vi "Set loggingEnabled.vi"(8 "error in (no error)":errorcluster, 10 "loggingEnabled":bool=TRUE, 11 "niDTS Comm String in":refnum<class "niDTS Comm String.lvclass">) -> (0 "error out":errorcluster, 3 "niDTS Comm String out":refnum<class "niDTS Comm String.lvclass">)   [LabVIEW 2015, in "niDTS CommLib.lvlib" / "niDTS Comm String.lvclass"]
uses:
  niDTS Comm String.lvclass
  niDTS Comm String.lvclass/niDTS Comm String.ctl
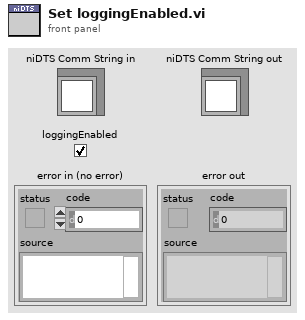
[diagram p1: front panel]
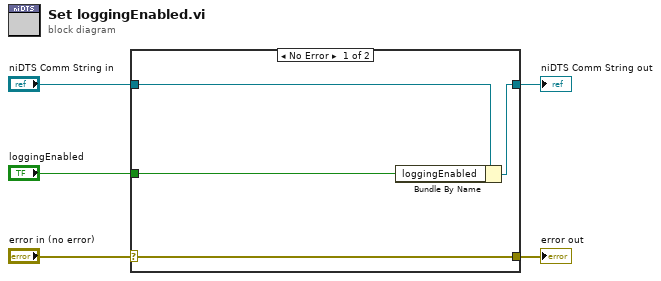
[diagram p0: block diagram]
diagram:
  n1 = case shown="No Error" "error in (no error)" {
    selector: "error in (no error)" -> [w9 w10]
    tunnel: [w9 w10] -> w4
    tunnel: [w7 w11] -> w2
    tunnel: "niDTS Comm String in" -> [w8 w11]
    tunnel: "loggingEnabled" -> [w6 _]
    frame No Error {
      n2 = Bundle By Name(cluster=w8, "loggingEnabled"=w6) -> (w7:refnum<class "niDTS Comm String.lvclass">)
    }
    frame Error {
    }
  }
  "error out" <- w4
  "niDTS Comm String out" <- w2
